vi "Tutorial.vi"() -> ()   [LabVIEW 2016]
panel:
  in  "Set Filter":bool
  out "OptionsFilterFreq2":string[][](array[string])
  out "OptionsFilterFreq1":string[][](array[string])
  in  "Read Filter Options":bool
  in  "3db Frequency #2":u16(ring) items=["100"]
  in  "3dB Frequency #1":u16(ring) items=["10"]
  in  "SampleCount":i64
  out "FilterType":string
  in  "Set Precision":bool
  in  "Precision":i32
  out "Info":string
  out "OptionsArray":string[][](array[string])
  in  "Property":string(combo)
  in  "Options":u16(ring)
  out "VariableInfos":string
  out "SelectedVarID":string
  in  "Write Project To Controller":bool
  in  "Set New Value":bool
  out "ControllerID":string
  in  "ReadOptions":bool
  in  "Network Devices":i32(listbox)=-1
  in  "ScanNetwork":bool
  in  "Variables":i32(listbox)=-1
  in  "ReadVariableIDs":bool
  in  "ReadController":bool
  out "error out":errorcluster
  # "GI.com is used to run a Network-Scan.\nLists all available Gantner-Devices\nin the Network with IP-Address\nand Location."
  # "Upload a device configuration (Q.station) into GI.config for further\nconfiguration. The result (on success) is a valid controller ID (needed \nfor later use)."
  # "Read VariableIDs + Infos from current\nproject in GI.config. IDs are necessary\nfor later use."
  # "Select a Variable to display Infos\nand to do further operations."
  # "This shows a simple example to set 1 variable property directly. \"Precision\" displays the actual setting of the selected variable. Using \"Set Precision\" a new setting can be applied."
  # "Depending on the Type of the selected variable, some more properties can be loaded (also with available options). Here, elements are only visible if an analog input is selected!\n\nUsing this example you can read properties of an analog input (see some examples in the drop-down list), and \"Set\" a new selected value."
  # "Read available options for the selected filter type. Use \"Set Filter\" to apply new settings."
  # "Using \"Write Project\" the current settings are checked for validation and transferred to the controller."
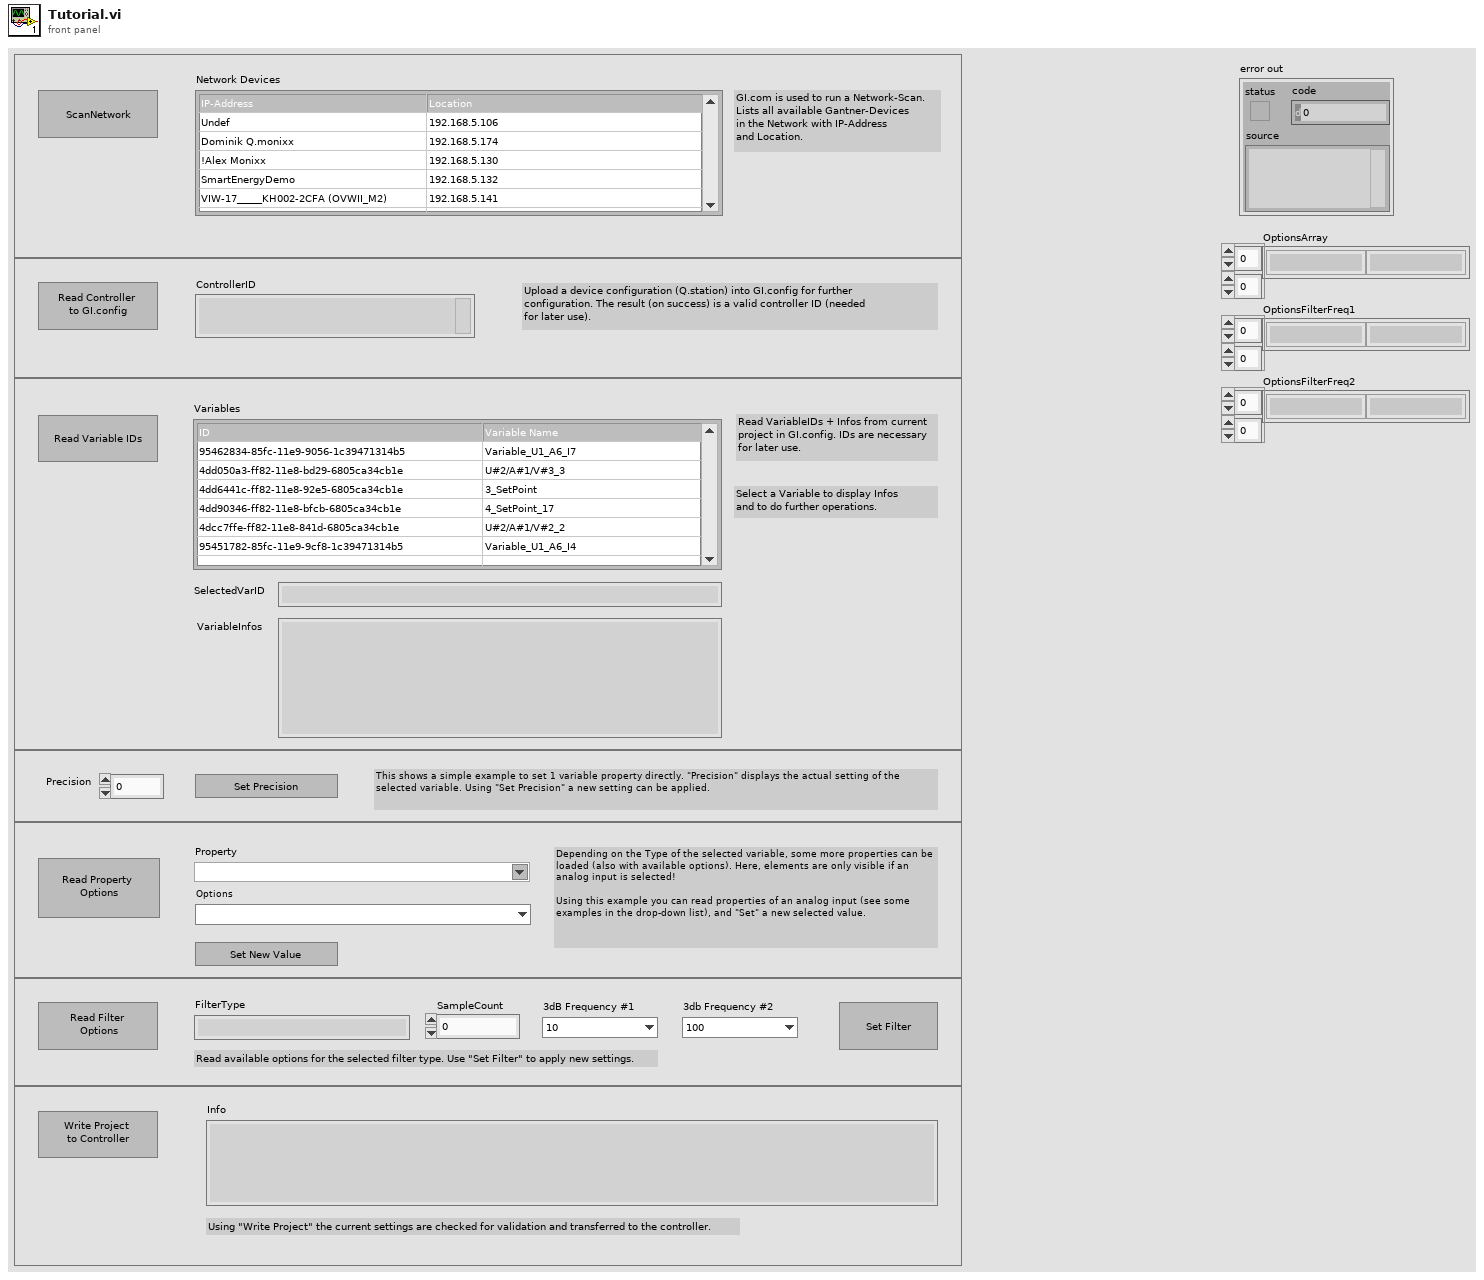
[diagram p1: front panel]
types:
  T1 = enum16{"idle", "idle2", "ScanNetwork", "ReadController", "ReadVarIDs", "ReadOptions", "SetConfig", "WriteToController", "SetPrecision", "ReadFilterOptions", "SetFilter"}
  T2 = enum16{"Bool", "Snippet", "Struct", "Int64", "Int32", "Float", "Double", "String"}
  T3 = typedef "VariableInfo.ctl" = cluster{"Name":string, "ID":string, "Type":string, "DataFormat":string, "DataDirection":string, "OwnerID":string, "AnalogInput Type":string, "Unit":string, "Precision":dbl, "Range":string, "FilterSettings":cluster{"Type":string, "SampleCount":i64, "3dB Frequency #1":string, "3dB Frequency #2":string, "TypeShort":string}}
  T4 = typedef "VariableArray.ctl" = cluster{"Array":T3[]}
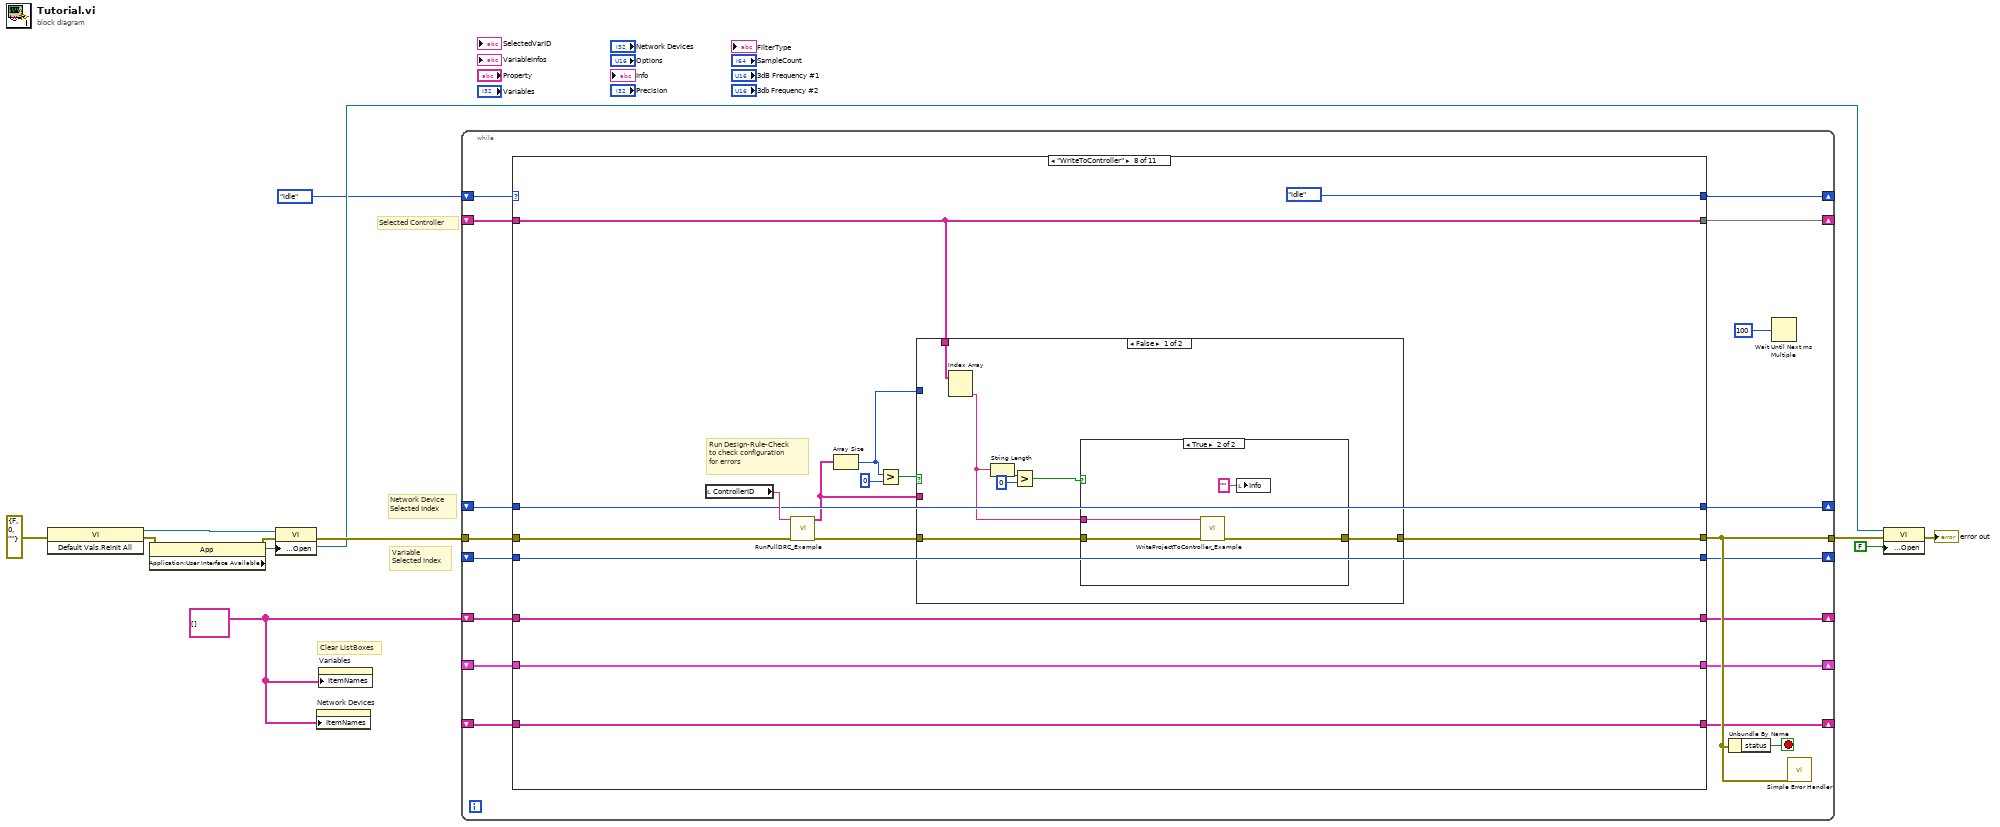
[diagram p0: block diagram]
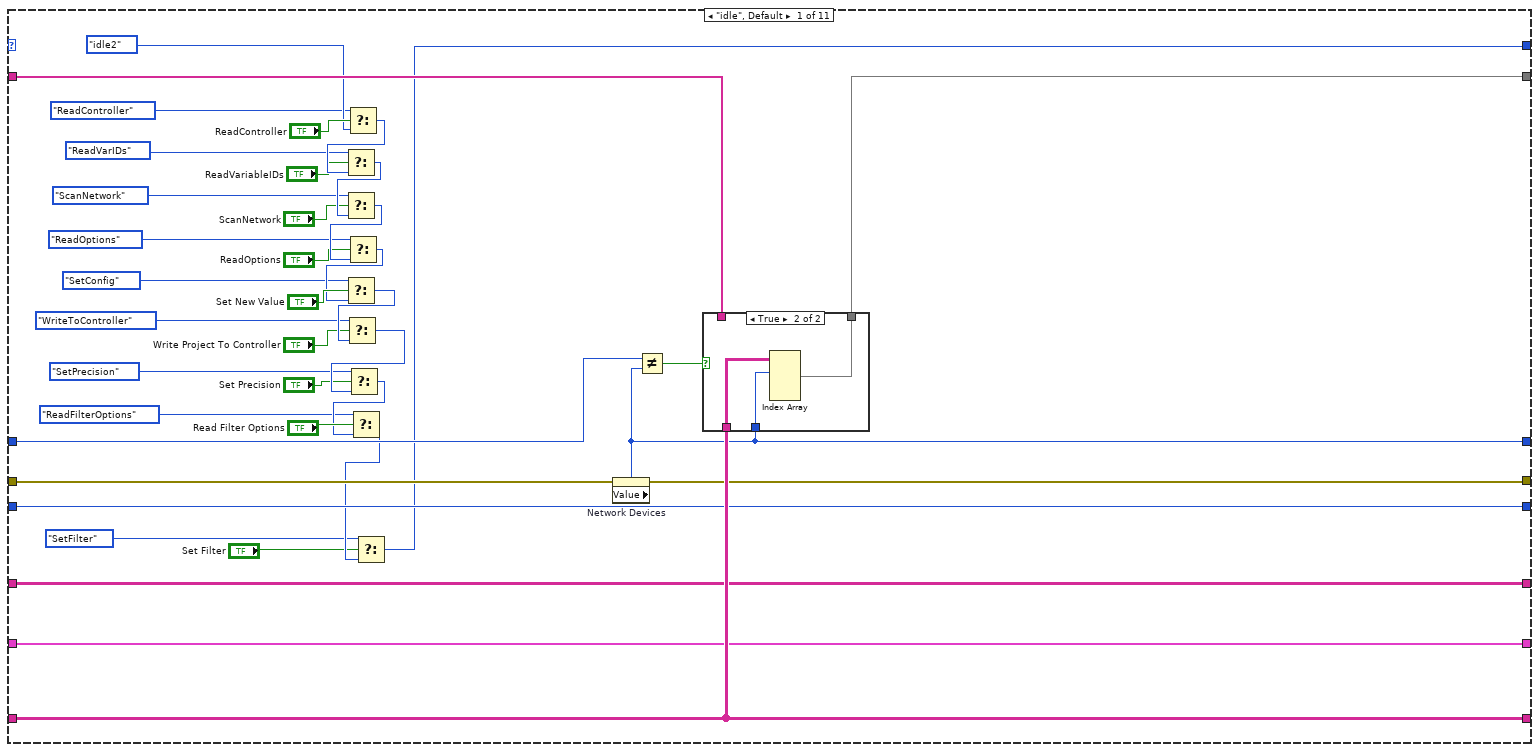
[diagram p2: hidden frame]
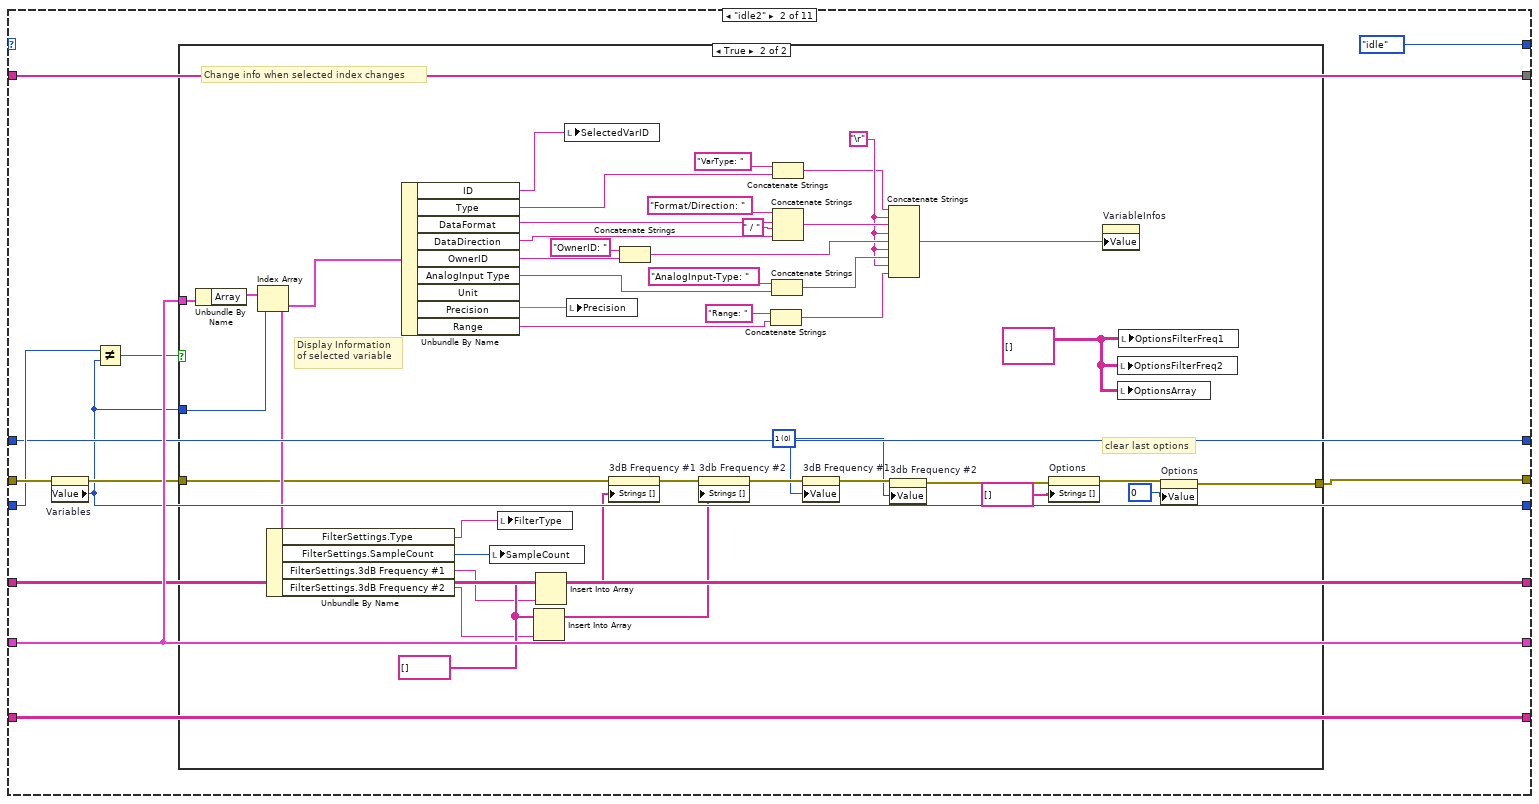
[diagram p4: hidden frame]
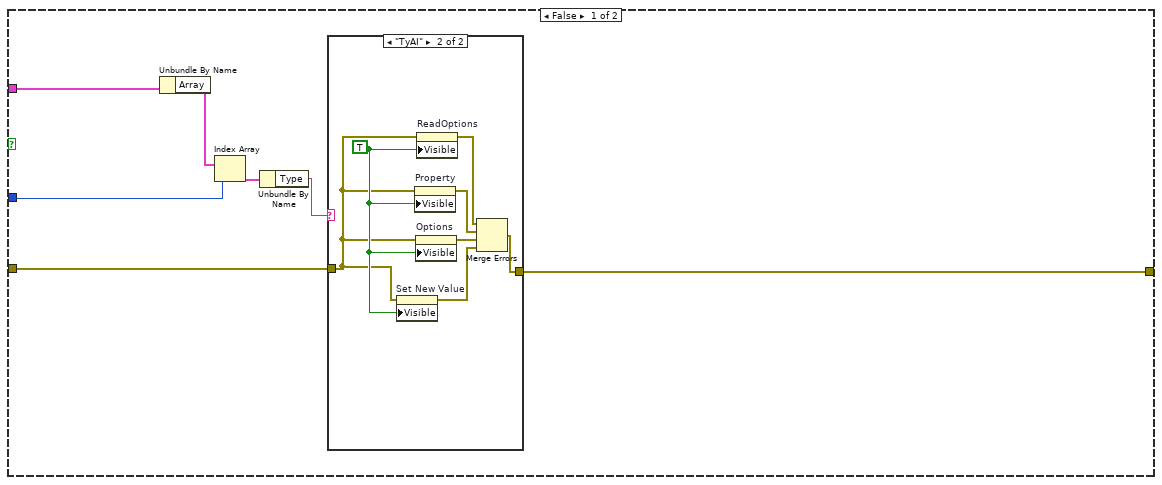
[diagram p5: hidden frame]
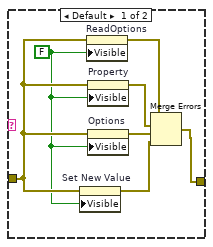
[diagram p6: hidden frame]
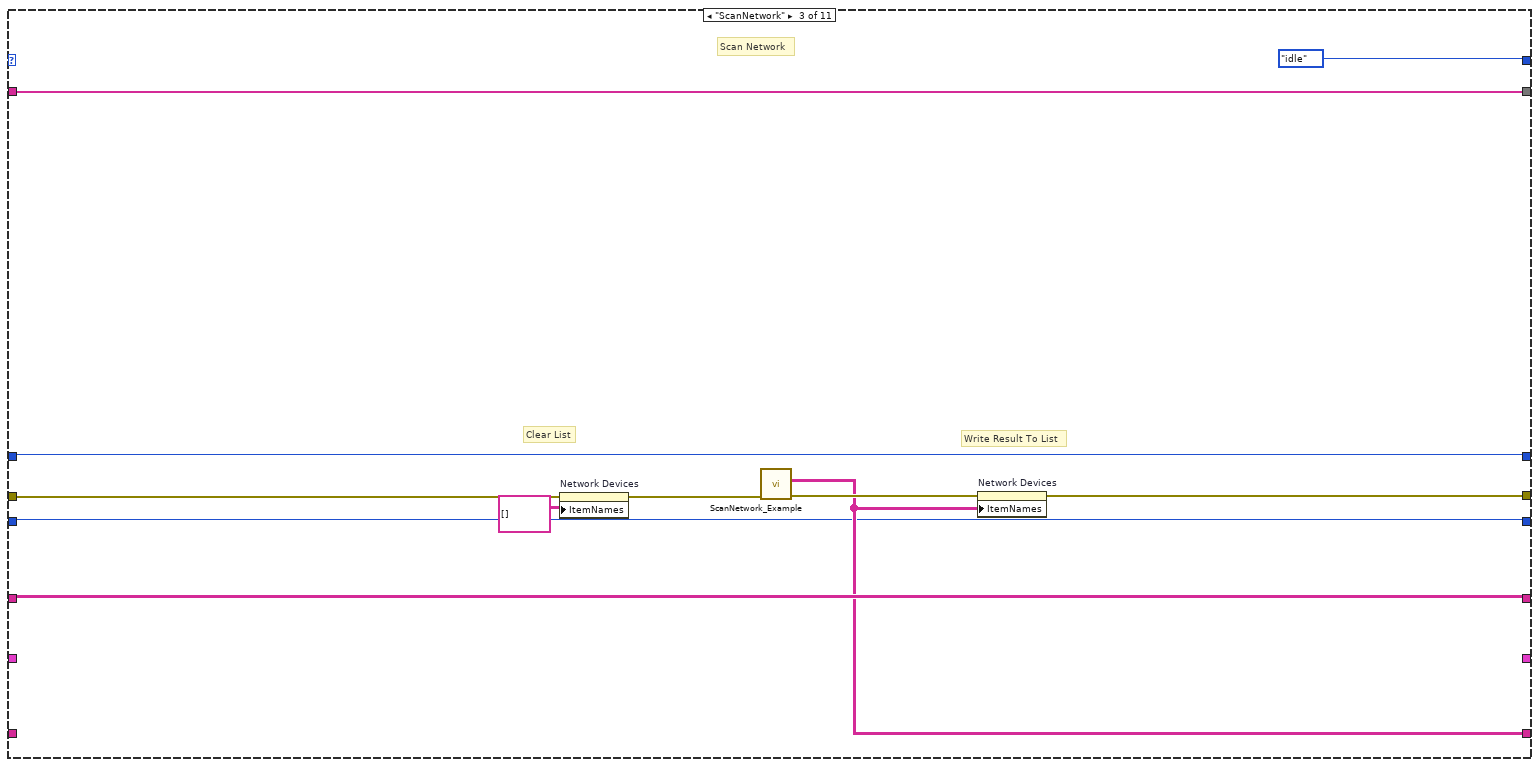
[diagram p7: hidden frame]
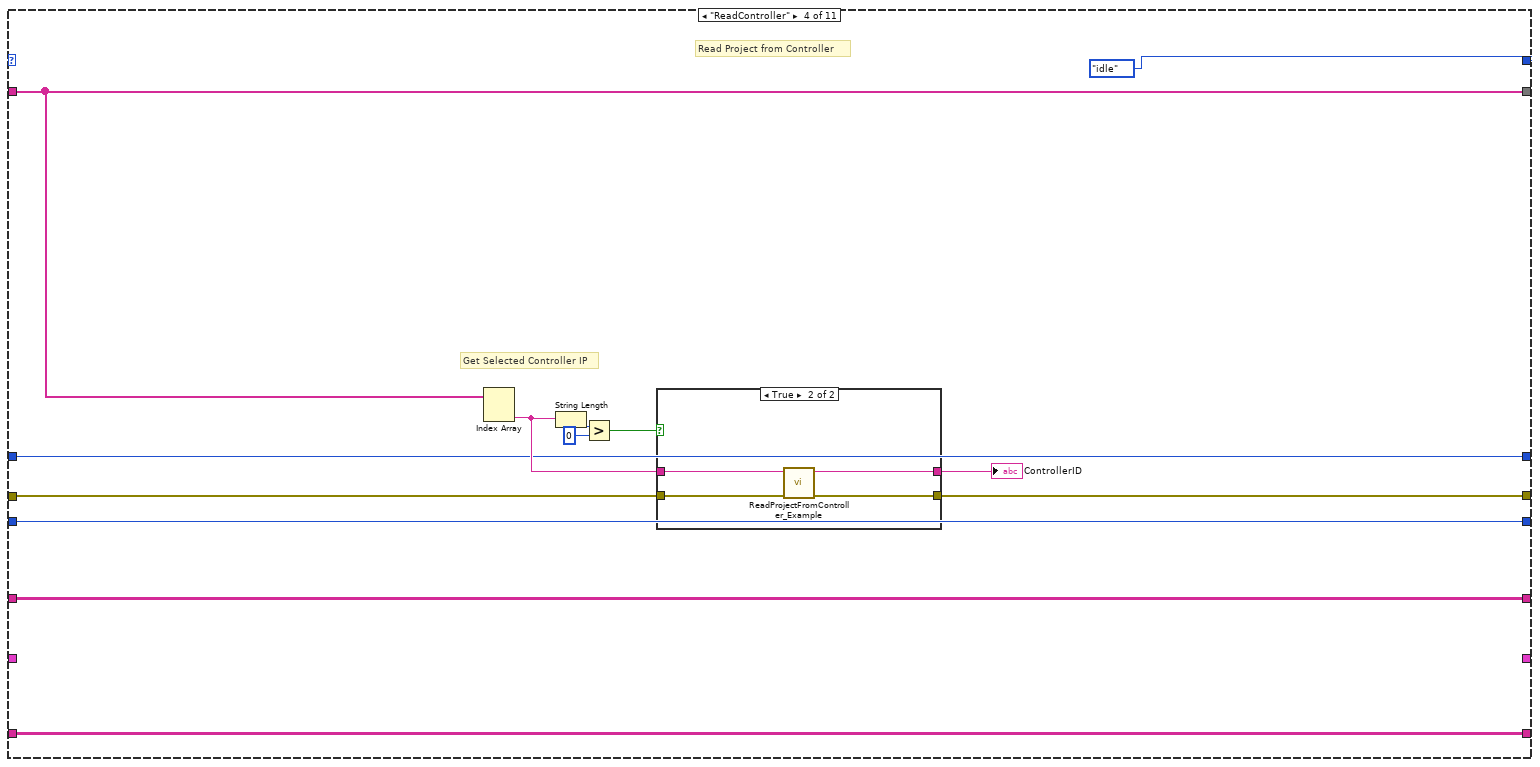
[diagram p8: hidden frame]
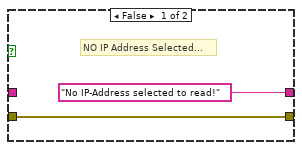
[diagram p9: hidden frame]
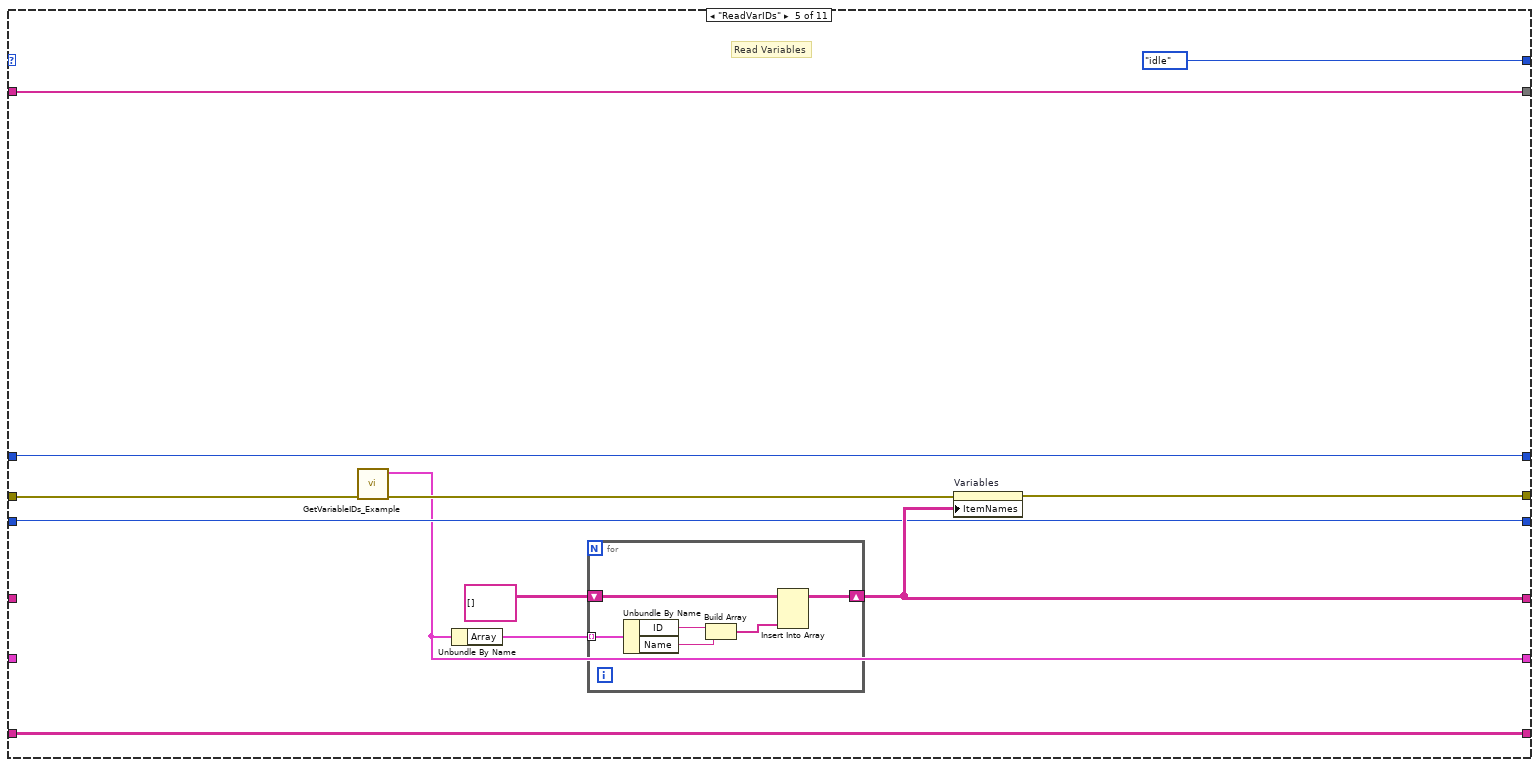
[diagram p10: hidden frame]
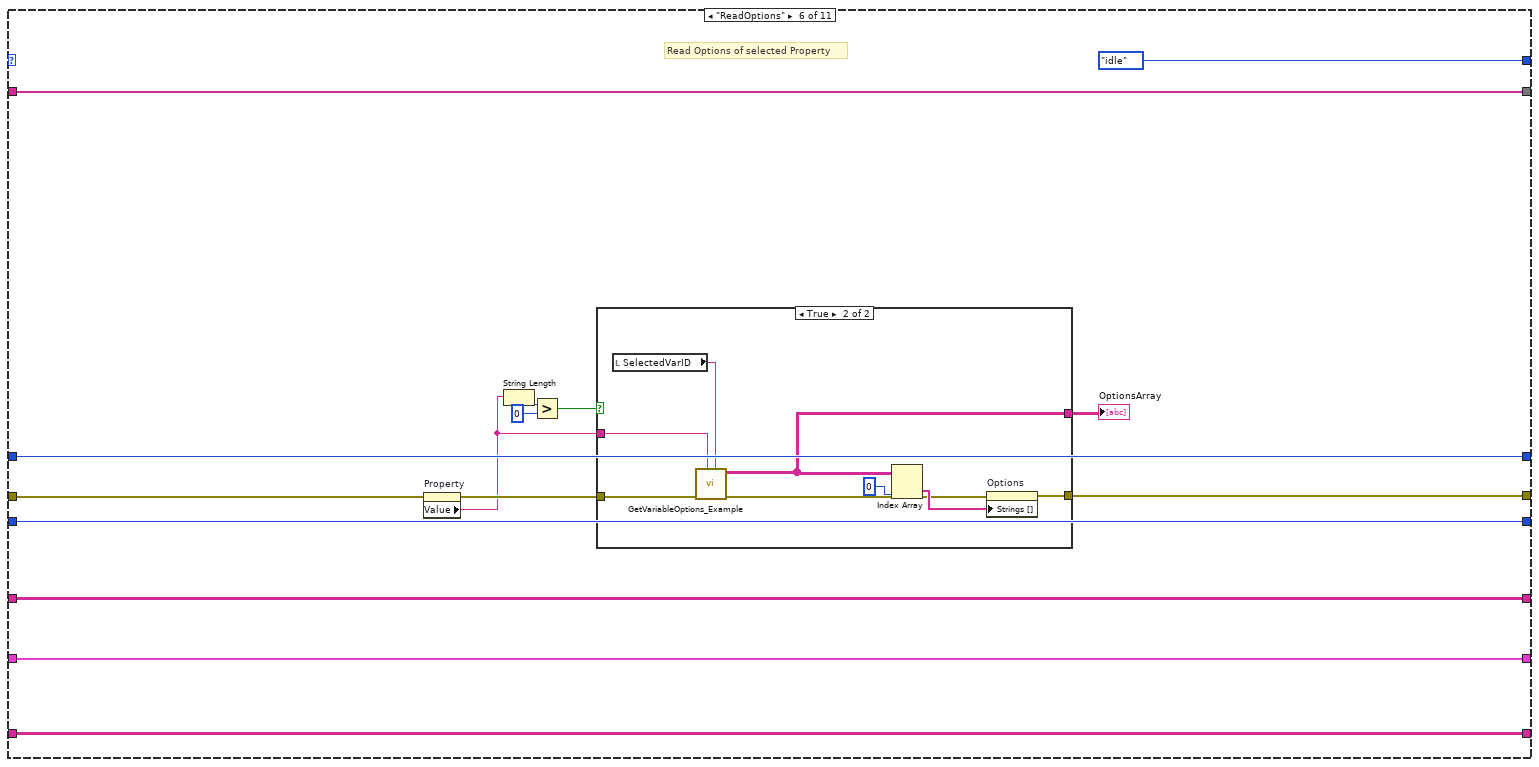
[diagram p11: hidden frame]
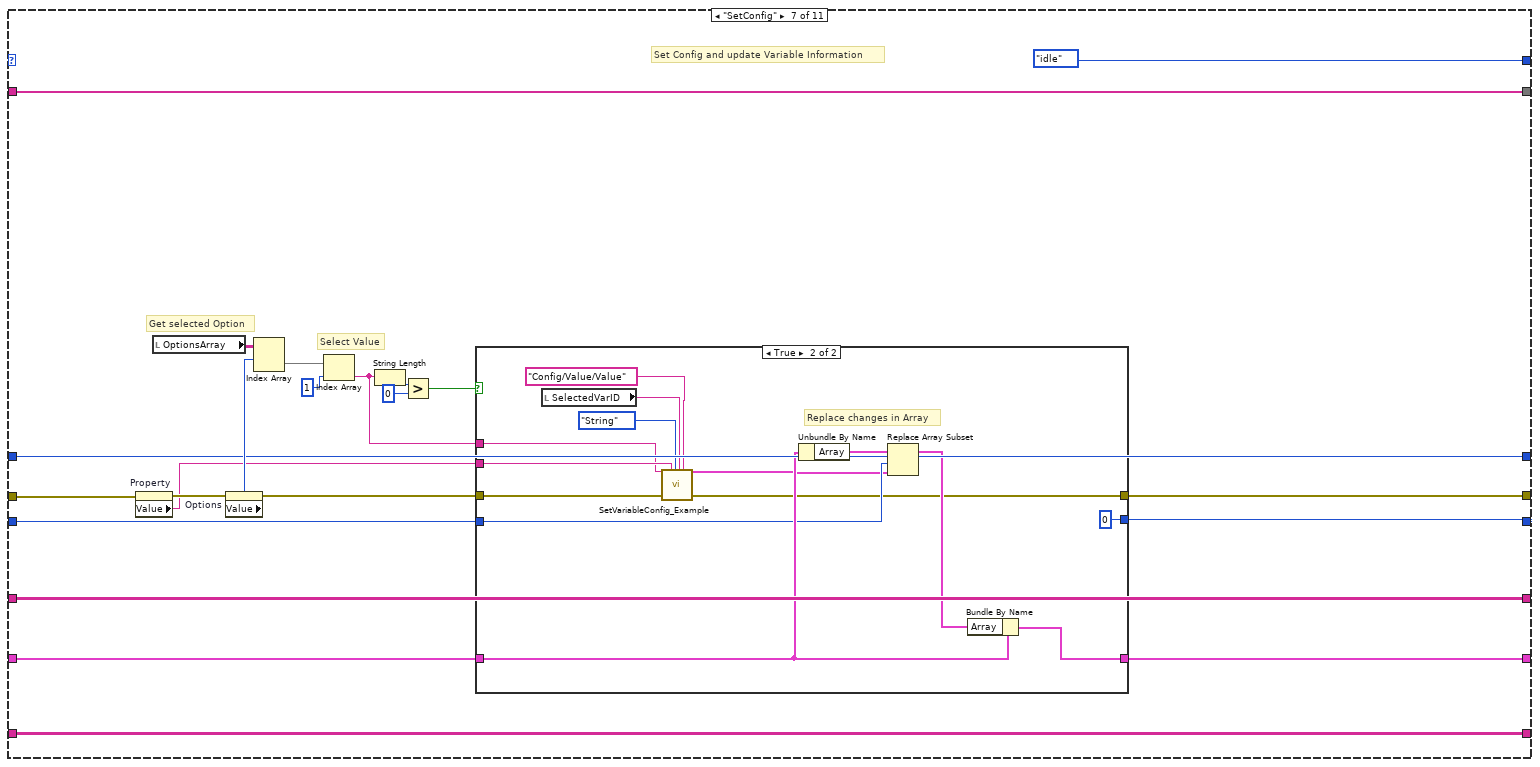
[diagram p13: hidden frame]
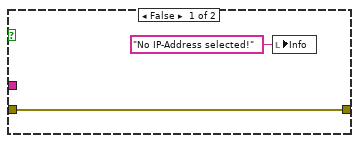
[diagram p15: hidden frame]
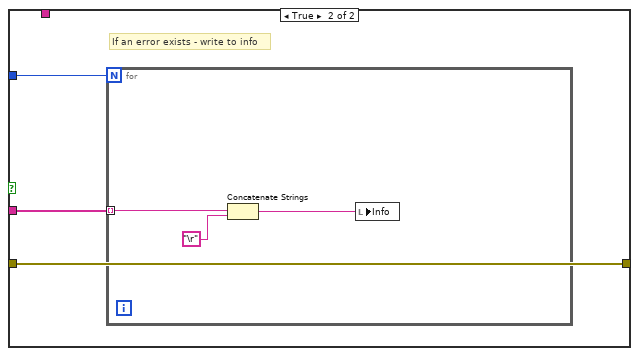
[diagram p16: hidden frame]
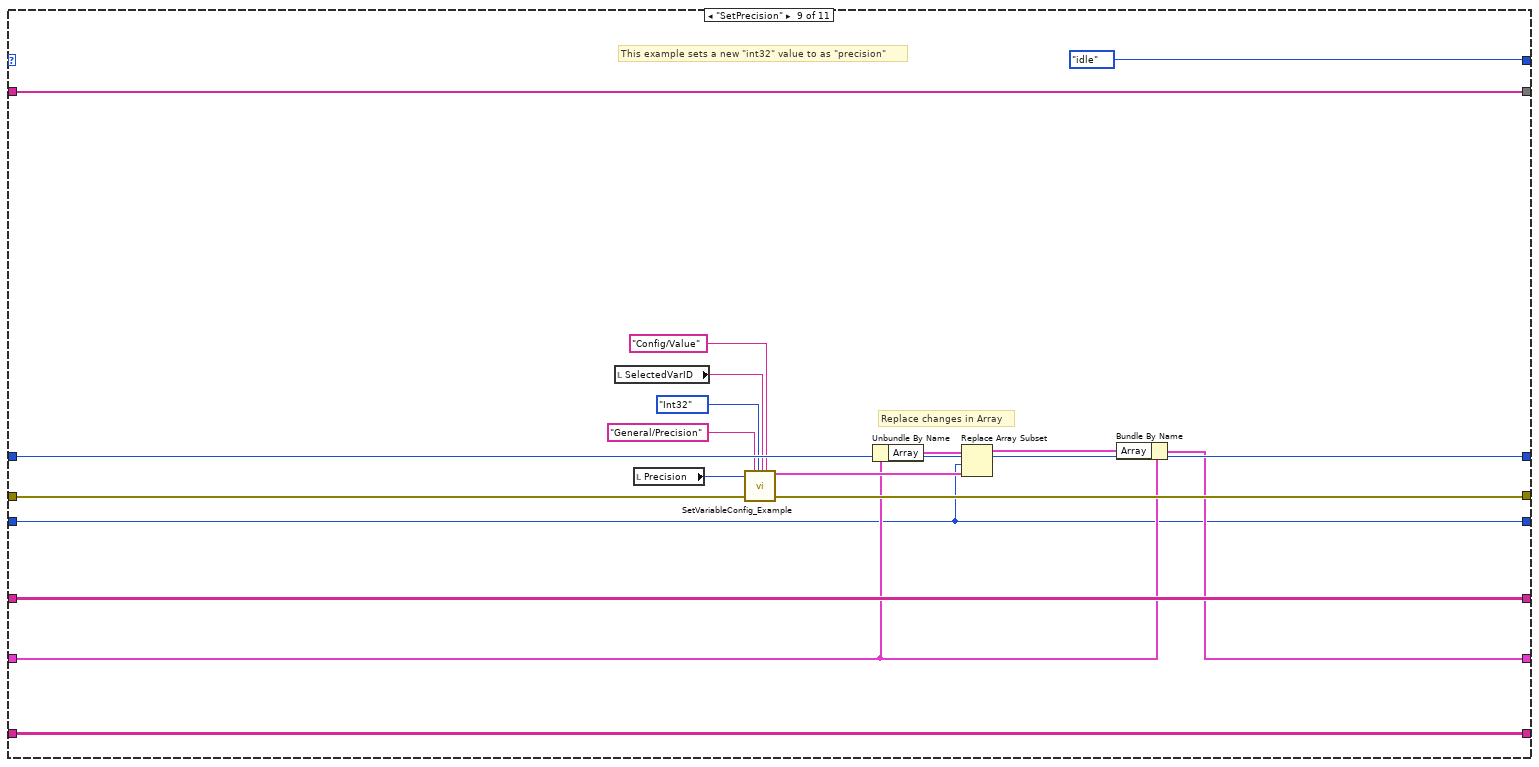
[diagram p17: hidden frame]
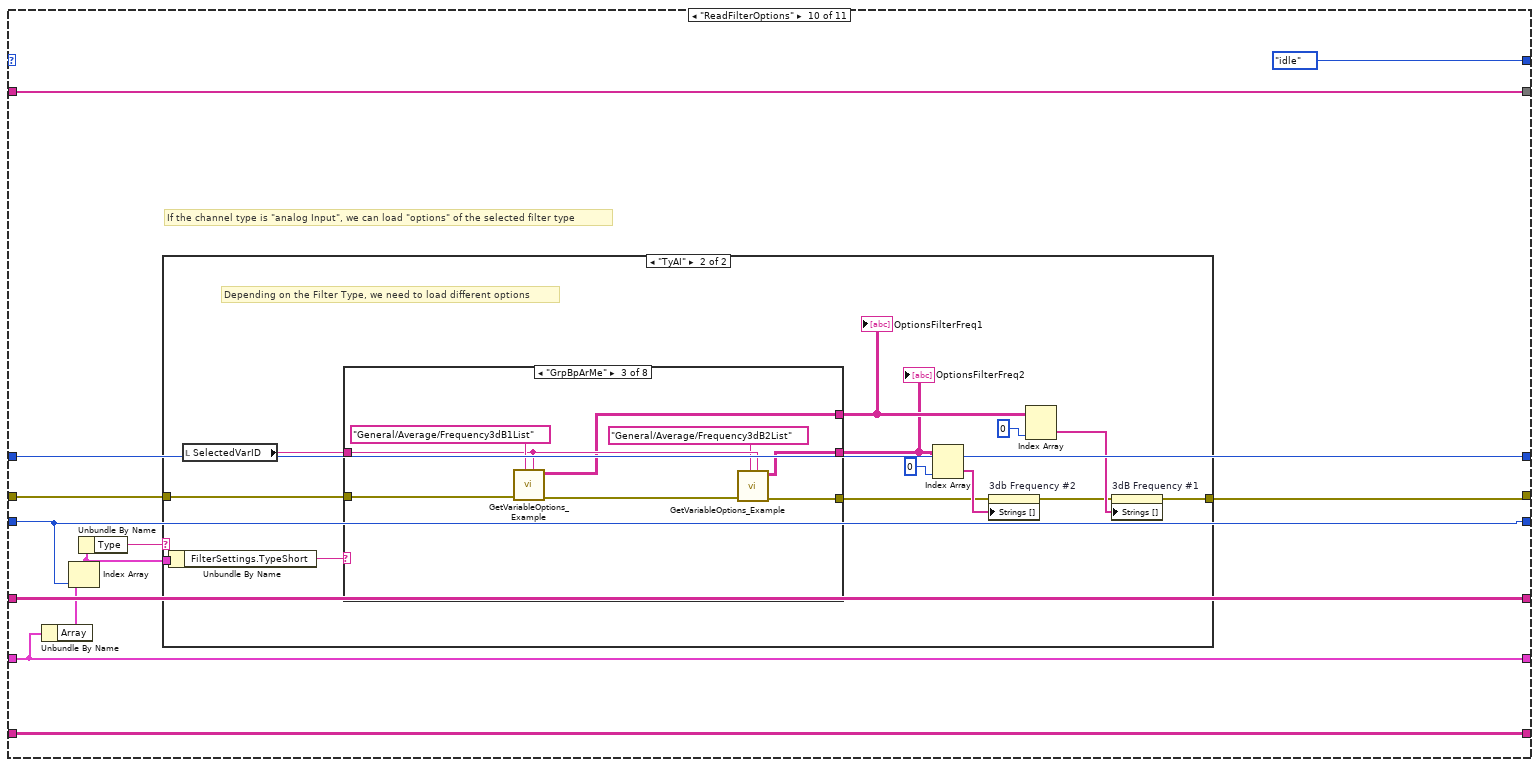
[diagram p18: hidden frame]
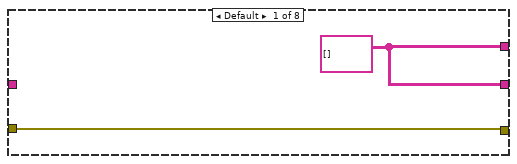
[diagram p20: hidden frame]
diagram:
  w2 = string[][] []
  # "Variable\nSelected Index"
  # "Network Device\nSelected Index"
  # "Selected Controller"
  # "Clear ListBoxes"
  n1 = invoke class="VI" method="Default Vals.Reinit All"(error in=errorcluster {"status"=FALSE, "code"=0, "source"=""} ("Fehler (Eingang, kein Fehler)")) -> (reference out=w12:refnum<vi>, error out=w10:errorcluster)  [unwired: 2 in, 1 out]
  n2 = property class="App"(error in=w10) -> (error out=w9:errorcluster, "Application:User Interface Available"=w11:bool)  [unwired: 1 in, 1 out]
  n3 = property class="VI"(reference=w12, error in=w9, "Front Panel.Open"=w11) -> (reference out=w3:refnum<vi>, error out=w7:errorcluster)
  n4 = property on="Network Devices" class="MCListbox (strict)"("ItemNames"=w2) -> ()  [unwired: 2 in, 2 out]
  n5 = property on="Variables" class="MCListbox (strict)"("ItemNames"=w2) -> ()  [unwired: 2 in, 2 out]
  n6 = while {
    tunnel: w7 -> [w29]
    tunnel: [w28] -> w4
    shift-right: [w14] -> _
    shift-left: T1."idle" -> [w13]
    shift-right: [w26] -> _
    shift-left: w2 -> [w27]
    shift-right: [w24] -> _
    shift-left: _ -> [w25]
    shift-right: [w23] -> _
    shift-left: _ -> [w22]
    shift-right: [w21] -> _
    shift-left: _ -> [w20]
    shift-right: [w19] -> _
    shift-left: _ -> [w18]
    shift-right: [w16] -> _
    shift-left: _ -> [w15]
    stop <- w17 stop-if-true
    n7 = case shown="\"WriteToController\"" w13 {
      tunnel: w29 -> [w64 w85 w156 w173 w190 w207 w237 w275 w308 w315 w389]
      tunnel: [w46 w76 w159 w172 w186 w208 w223 w265 w307 w314 w387] -> w28
      tunnel: w27 -> [w56 w81 w160 w171 _ w212 w242 w273 w310 w323 w394]
      tunnel: [w56 w81 w160 w171 w185 w212 w242 w273 w310 w323 w394] -> w26
      tunnel: w25 -> [w61 w80 _ w170 w191 w211 w243 w272 w309 w324 w395]
      tunnel: [w61 w80 w157 w170 w191 w211 w243 w272 w309 w324 w395] -> w24
      tunnel: [w55 w79 w152 w163 w183 w204 w238 w269 w311 w319 w393] -> w23
      tunnel: w22 -> [w63 w79 w152 w163 w183 w204 w238 w269 w311 w319 w393]
      tunnel: [w60 w78 w151 w162 w181 w203 w239 w264 w312 w318 w392] -> w21
      tunnel: w20 -> [w59 w78 w151 w162 w181 w203 w239 w264 w312 w318 w392]
      tunnel: [w47 w75 w153 w164 w184 w205 w224 w270 w296 w320 0 ("Value")] -> w19
      tunnel: w18 -> [w47 w84 w153 w164 w184 w205 w226 w270 w296 w320 w384]
      tunnel: [w50 w83 _ _ w182 w210 w227 w271 w297 w322 w385] -> w16
      tunnel: w15 -> [w50 w83 _ _ _ w210 w225 w271 w298 w322 w386]
      tunnel: [w33 T1."idle" T1."idle" T1."idle" T1."idle" T1."idle" T1."idle" T1."idle" T1."idle" T1."idle" T1."idle"] -> w14
      frame "idle", Default {
        n8 = Select(t=T1."ReadController", s="ReadController", f=T1."idle2") -> (s? t:f=w68:T1)
        n9 = Select(t=T1."ReadVarIDs", s="ReadVariableIDs", f=w68) -> (s? t:f=w66:T1)
        n10 = Select(t=T1."ScanNetwork", s="ScanNetwork", f=w66) -> (s? t:f=w58:T1)
        n11 = Select(t=T1."ReadOptions", s="ReadOptions", f=w58) -> (s? t:f=w53:T1)
        n12 = Select(t=T1."SetConfig", s="Set New Value", f=w53) -> (s? t:f=w52:T1)
        n13 = Select(t=T1."WriteToController", s="Write Project To Controller", f=w52) -> (s? t:f=w49:T1)
        n14 = Select(t=T1."SetPrecision", s="Set Precision", f=w49) -> (s? t:f=w44:T1)
        n15 = Select(t=T1."ReadFilterOptions", s="Read Filter Options", f=w44) -> (s? t:f=w34:T1)
        n16 = Select(t=T1."SetFilter", s="Set Filter", f=w34) -> (s? t:f=w33:T1)
        n17 = property on="Network Devices" class="MCListbox (strict)"(error in=w64) -> (error out=w46:errorcluster, "Value"=w55:i32)  [unwired: 1 in, 1 out]
        n18 = Not Equal?(x=w63, y=w55) -> (x != y?=w62:bool)
        n19 = case shown="True" w62 {
          tunnel: w55 -> [_ w71]
          tunnel: w61 -> [_ w73]
          tunnel: [w70 w72] -> w60
          tunnel: w59 -> [w70 _]
          frame False {
          }
          frame True {
            n20 = Index Array(array=w73, index (row) #1=w71) -> (element #1=w72:string[])  [unwired: 3 in, 1 out]
          }
        }
      }
      frame "idle2" {
        n21 = property on="Variables" class="MCListbox (strict)"(error in=w85) -> (error out=w77:errorcluster, "Value"=w75:i32)  [unwired: 1 in, 1 out]
        n22 = Not Equal?(x=w84, y=w75) -> (x != y?=w82:bool)
        n23 = case shown="True" w82 {
          tunnel: w75 -> [w90 w149]
          tunnel: w83 -> [w91 w148]
          tunnel: w77 -> [w87 w119]
          tunnel: [w86 w111] -> w76
          frame False {
            n24 = Unbundle By Name(w91) -> ("Array"=w92:T3[])
            n25 = Index Array(array=w92, index=w90) -> (element=w89:T3)
            n26 = Unbundle By Name(w89) -> ("Type"=w88:string)
            n27 = case shown="\"TyAI\"" w88 {
              tunnel: w87 -> [w95 w100]
              tunnel: [w96 w103] -> w86
              frame Default {
                w93 = FALSE ("Visible")
                n28 = property on="Set New Value" class="Bool"(error in=w95, "Visible"=w93) -> (error out=w94:errorcluster)  [unwired: 1 in, 1 out]
                n29 = property on="ReadOptions" class="Bool"(error in=w95, "Visible"=w93) -> (error out=w97:errorcluster)  [unwired: 1 in, 1 out]
                n30 = property on="Property" class="CmbBox"(error in=w95, "Visible"=w93) -> (error out=w98:errorcluster)  [unwired: 1 in, 1 out]
                n31 = property on="Options" class="Ring (strict)"(error in=w95, "Visible"=w93) -> (error out=w99:errorcluster)  [unwired: 1 in, 1 out]
                n32 = Merge Errors(w97, w98, w99, w94) -> (w96:errorcluster)
              }
              frame "TyAI" {
                w102 = TRUE ("Visible")
                n33 = property on="Set New Value" class="Bool"(error in=w100, "Visible"=w102) -> (error out=w101:errorcluster)  [unwired: 1 in, 1 out]
                n34 = property on="Property" class="CmbBox"(error in=w100, "Visible"=w102) -> (error out=w105:errorcluster)  [unwired: 1 in, 1 out]
                n35 = property on="Options" class="Ring (strict)"(error in=w100, "Visible"=w102) -> (error out=w106:errorcluster)  [unwired: 1 in, 1 out]
                n36 = property on="ReadOptions" class="Bool"(error in=w100, "Visible"=w102) -> (error out=w104:errorcluster)  [unwired: 1 in, 1 out]
                n37 = Merge Errors(w104, w105, w106, w101) -> (w103:errorcluster)
              }
            }
          }
          frame True {
            w107 = u16 0 items=["1"] ("3dB Frequency #1")
            w122 = string[] [] ("Strings []")
            w114 = string[][] [] ("Strings []")
            w112 = u16 0 items=[""] ("Options")
            w128 = "\r"
            # "clear last options"
            # "Change info when selected index changes"
            # "Display Information\nof selected variable"
            n38 = Unbundle By Name(w148) -> ("Array"=w147:T3[])
            n39 = Index Array(array=w147, index=w149) -> (element=w143:T3)
            n40 = Unbundle By Name(w143) -> ("FilterSettings.Type"=w124:string, "FilterSettings.SampleCount"=w123:i64, "FilterSettings.3dB Frequency #1"=w121:string, "FilterSettings.3dB Frequency #2"=w120:string)
            n41 = Unbundle By Name(w143) -> ("ID"=w145:string, "Type"=w141:string, "DataFormat"=w139:string, "DataDirection"=w137:string, "OwnerID"=w135:string, "AnalogInput Type"=w131:string, "Precision"=w144:dbl, "Range"=w126:string)  [unwired: 1 out]
            n42 = local write "SampleCount"(w123) -> ()
            n43 = local write "FilterType"(w124) -> ()
            n44 = Insert Into Array(array=w122, new element=w120) -> (w116:string[])  [unwired: 1 in]
            n45 = Insert Into Array(array=w122, new element=w121) -> (w117:string[])  [unwired: 1 in]
            n46 = local write "SelectedVarID"(w145) -> ()
            n47 = local write "Precision"(w144) -> ()
            n48 = property on="3dB Frequency #1" class="Ring (strict)"(error in=w119, "Strings []"=w117) -> (error out=w118:errorcluster)  [unwired: 1 in, 1 out]
            n49 = Concatenate Strings("OwnerID: " ("string"), w135) -> (w133:string)
            n50 = property on="3db Frequency #2" class="Ring (strict)"(error in=w118, "Strings []"=w116) -> (error out=w110:errorcluster)  [unwired: 1 in, 1 out]
            n51 = Concatenate Strings("Range: " ("string"), w126) -> (w125:string)
            n52 = Concatenate Strings("AnalogInput-Type: " ("string"), w131) -> (w130:string)
            n53 = Concatenate Strings("VarType: " ("string"), w141) -> (w115:string)
            n54 = Concatenate Strings("Format/Direction: " ("string"), w139, " / " ("string"), w137) -> (w134:string)
            n55 = property on="3dB Frequency #1" class="Ring (strict)"(error in=w110, "Value"=w107) -> (error out=w109:errorcluster)  [unwired: 1 in, 1 out]
            n56 = Concatenate Strings(w115, w128, w134, w128, w133, w128, w130, w128, w125) -> (w129:string)
            n57 = property on="3db Frequency #2" class="Ring (strict)"(error in=w109, "Value"=w107) -> (error out=w108:errorcluster)  [unwired: 1 in, 1 out]
            n58 = property on="Options" class="Ring (strict)"(error in=w108, "Strings []"=string[] []) -> (error out=w146:errorcluster)  [unwired: 1 in, 1 out]
            n59 = property on="VariableInfos" class="Str"("Value"=w129) -> ()  [unwired: 2 in, 2 out]
            n60 = local write "OptionsFilterFreq2"(w114) -> ()
            n61 = local write "OptionsArray"(w114) -> ()
            n62 = local write "OptionsFilterFreq1"(w114) -> ()
            n63 = property on="Options" class="Ring (strict)"(error in=w146, "Value"=w112) -> (error out=w111:errorcluster)  [unwired: 1 in, 1 out]
          }
        }
      }
      frame "ScanNetwork" {
        # "Write Result To List"
        # "Clear List"
        # "Scan Network"
        n64 = property on="Network Devices" class="MCListbox (strict)"(error in=w156, "ItemNames"=string[][] [] ("Item Names")) -> (error out=w155:errorcluster)  [unwired: 1 in, 1 out]
        n65 = call "ScanNetwork_Example.vi"("Fehler (Eingang, kein Fehler)"=w155) -> ("Fehler (Ausgang)"=w158:errorcluster, "NetworkDevices Array"=w157:string[][])  [unwired: 9 in]
        n66 = property on="Network Devices" class="MCListbox (strict)"(error in=w158, "ItemNames"=w157) -> (error out=w159:errorcluster)  [unwired: 1 in, 1 out]
      }
      frame "ReadController" {
        # "Get Selected Controller IP"
        # "Read Project from Controller"
        n67 = Index Array(array=w162) -> (element #2=w165:string)  [unwired: 2 in, 1 out]
        n68 = String Length(string=w165) -> (length=w169:i32)
        n69 = Greater?(x=w169, y=0) -> (0:w167:bool)
        n70 = case shown="True" w167 {
          tunnel: w173 -> [w175 w179]
          tunnel: [w175 w178] -> w172
          tunnel: w165 -> [_ w177]
          tunnel: ["No IP-Address selected to read!" ("standard output") w176] -> w166
          frame False {
            # "NO IP Address Selected..."
          }
          frame True {
            n71 = call "ReadProjectFromController_Example.vi"("Fehler (Eingang, kein Fehler)"=w179, "ControllerIP"=w177) -> ("Fehler (Ausgang)"=w178:errorcluster, "ControllerID"=w176:string)  [unwired: 8 in]
          }
        }
        "ControllerID" <- w166
      }
      frame "ReadVarIDs" {
        # "Read Variables"
        n72 = call "GetVariableIDs_Example.vi"("Fehler (Eingang, kein Fehler)"=w190) -> ("Fehler (Ausgang)"=w189:errorcluster, "VariableArray out"=w182:T4)  [unwired: 9 in]
        n73 = Unbundle By Name(w182) -> ("Array"=w188:T3[])
        n74 = for {
          tunnel: w188 -> [w197] mode=indexing
          shift-right: [w195] -> w185
          shift-left: string[][] [] ("Item Names") -> [w196]
          n75 = Unbundle By Name(w197) -> ("ID"=w194:string, "Name"=w193:string)
          n76 = Build Array(w194, w193) -> (w192:string[])
          n77 = Insert Into Array(array=w196, new element=w192) -> (w195:string[][])  [unwired: 2 in]
        }
        n78 = property on="Variables" class="MCListbox (strict)"(error in=w189, "ItemNames"=w185) -> (error out=w186:errorcluster)  [unwired: 1 in, 1 out]
      }
      frame "ReadOptions" {
        # "Read Options of selected Property"
        n79 = property on="Property" class="CmbBox"(error in=w207) -> (error out=w206:errorcluster, "Value"=w199:string)  [unwired: 1 in, 1 out]
        n80 = String Length(string=w199) -> (length=w202:i32)
        n81 = Greater?(x=w202, y=0) -> (0:w200:bool)
        n82 = case shown="True" w200 {
          tunnel: [_ w221] -> w209
          tunnel: [w213 w217] -> w208
          tunnel: w206 -> [w213 w216]
          tunnel: w199 -> [_ w215]
          frame False {
          }
          frame True {
            n83 = local read "SelectedVarID"() -> (w214:string)
            n84 = call "GetVariableOptions_Example.vi"("VariableID"=w214, "PropertyName"=w215, "Fehler (Eingang, kein Fehler)"=w216) -> ("Fehler (Ausgang)"=w218:errorcluster, "Options"=w221:string[][])  [unwired: 7 in]
            n85 = Index Array(array=w221, index (col)=0 ("disabled index (col)")) -> (element=w219:string[])  [unwired: 1 in]
            n86 = property on="Options" class="Ring (strict)"(error in=w218, "Strings []"=w219) -> (error out=w217:errorcluster)  [unwired: 1 in, 1 out]
          }
        }
        "OptionsArray" <- w209
      }
      frame "SetConfig" {
        # "Set Config and update Variable Information"
        # "Select Value"
        # "Get selected Option"
        n87 = property on="Property" class="CmbBox"(error in=w237) -> (error out=w236:errorcluster, "Value"=w228:string)  [unwired: 1 in, 1 out]
        n88 = local read "OptionsArray"() -> (w241:string[][])
        n89 = property on="Options" class="Ring (strict)"(error in=w236) -> (error out=w230:errorcluster, "Value"=w240:u16)  [unwired: 1 in, 1 out]
        n90 = Index Array(array=w241, index (row)=w240) -> (element=w233:string[])  [unwired: 1 in]
        n91 = Index Array(array=w233, index=1) -> (element=w229:string)
        n92 = String Length(string=w229) -> (length=w235:i32)
        n93 = Greater?(x=w235, y=0) -> (0:w232:bool)
        n94 = case shown="True" w232 {
          tunnel: w230 -> [w246 w253]
          tunnel: [w246 w254] -> w223
          tunnel: w229 -> [_ w250]
          tunnel: w228 -> [_ w252]
          tunnel: [w244 w258] -> w227
          tunnel: w226 -> [w245 w256]
          tunnel: w225 -> [w244 w257]
          tunnel: [w245 0 ("Value")] -> w224
          frame False {
          }
          frame True {
            # "Replace changes in Array"
            n95 = local read "SelectedVarID"() -> (w251:string)
            n96 = call "SetVariableConfig_Example.vi"("StringValue or Snippet 2"=w250, "Fehler (Eingang, kein Fehler)"=w253, "PropertyName"=w252, "DataType"=T2."String", "VariableID"=w251, "ConfigMemberName"="Config/Value/Value" ("MemberName")) -> ("VariableInfo out"=w255:T3, "Fehler (Ausgang)"=w254:errorcluster)  [unwired: 20 in]
            n97 = Unbundle By Name(w257) -> ("Array"=w260:T3[])
            n98 = Replace Array Subset(array=w260, new element=w255, index=w256) -> (w259:T3[])
            n99 = Bundle By Name(cluster=w257, "Array"=w259) -> (w258:T4)
          }
        }
      }
      frame "WriteToController" {
        # "Run Design-Rule-Check\nto check configuration\nfor errors"
        n100 = local read "ControllerID"() -> (w274:string)
        n101 = call "RunFullDRC_Example.vi"("Fehler (Eingang, kein Fehler)"=w275, "ControllerID"=w274) -> ("Fehler (Ausgang)"=w266:errorcluster, "Results"=w262:string[])  [unwired: 8 in]
        n102 = Array Size(array=w262) -> (size(s)=w263:i32)
        n103 = Greater?(x=w263, y=0) -> (0:w267:bool)
        n104 = case shown="False" w267 {
          tunnel: w266 -> [w282 w291]
          tunnel: [w281 w291] -> w265
          tunnel: w264 -> [w280 _]
          tunnel: w263 -> [_ w290]
          tunnel: w262 -> [_ w289]
          frame False {
            n105 = Index Array(array=w280) -> (element #2=w276:string)  [unwired: 2 in, 1 out]
            n106 = String Length(string=w276) -> (length=w279:i32)
            n107 = Greater?(x=w279, y=0) -> (0:w277:bool)
            n108 = case shown="True" w277 {
              tunnel: w282 -> [w284 w288]
              tunnel: [w284 w287] -> w281
              tunnel: w276 -> [_ w286]
              frame False {
                n109 = local write "Info"("No IP-Address selected!" ("Info")) -> ()
              }
              frame True {
                n110 = call "WriteProjectToController_Example.vi"("Fehler (Eingang, kein Fehler)"=w288, "Controller IP"=w286) -> ("Fehler (Ausgang)"=w287:errorcluster)  [unwired: 9 in]
                n111 = local write "Info"("" ("Info")) -> ()
              }
            }
          }
          frame True {
            # "If an error exists - write to info"
            n112 = for {
              N: w290 -> [_]
              tunnel: w289 -> [w294] mode=indexing
              n113 = Concatenate Strings(w294, "\r") -> (w292:string)
              n114 = local write "Info"(w292) -> ()
            }
          }
        }
      }
      frame "SetPrecision" {
        # "This example sets a new \"int32\" value to as \"precision\""
        # "Replace changes in Array"
        n115 = local read "SelectedVarID"() -> (w306:string)
        n116 = local read "Precision"() -> (w304:i32)
        n117 = call "SetVariableConfig_Example.vi"("Int32Value or struct"=w304, "Fehler (Eingang, kein Fehler)"=w308, "PropertyName"="General/Precision", "DataType"=T2."Int32", "VariableID"=w306, "ConfigMemberName"="Config/Value" ("MemberName")) -> ("VariableInfo out"=w300:T3, "Fehler (Ausgang)"=w307:errorcluster)  [unwired: 20 in]
        n118 = Unbundle By Name(w298) -> ("Array"=w301:T3[])
        n119 = Replace Array Subset(array=w301, new element=w300, index=w296) -> (w299:T3[])
        n120 = Bundle By Name(cluster=w298, "Array"=w299) -> (w297:T4)
      }
      frame "ReadFilterOptions" {
        # "If the channel type is \"analog Input\", we can load \"options\" of the selected filter type"
        n121 = Unbundle By Name(w322) -> ("Array"=w321:T3[])
        n122 = Index Array(array=w321, index=w320) -> (element=w316:T3)
        n123 = Unbundle By Name(w316) -> ("Type"=w317:string)
        n124 = case shown="\"TyAI\"" w317 {
          tunnel: w316 -> [_ w337]
          tunnel: w315 -> [w325 w335]
          tunnel: [w325 w326] -> w314
          frame Default {
          }
          frame "TyAI" {
            # "Depending on the Filter Type, we need to load different options"
            n125 = Unbundle By Name(w337) -> ("FilterSettings.TypeShort"=w336:string)
            n126 = local read "SelectedVarID"() -> (w338:string)
            n127 = case shown="\"GrpBpArMe\"" w336 {
              tunnel: w338 -> [_ _ w346 w355 w360 w365 w371 w375]
              tunnel: w335 -> [w340 w342 w350 w354 w362 w367 w373 w380]
              tunnel: [w340 w342 w347 w353 w359 w366 w372 w378] -> w328
              tunnel: [w339 w341 w344 string[][] [] ("Options") string[][] [] ("Options") string[][] [] ("Options") string[][] [] ("Options") w377] -> w331
              tunnel: [w339 w341 w343 w352 w358 w363 w370 w376] -> w332
              frame Default {
                w339 = string[][] [] ("Options")
              }
              frame "GrpNo" {
                w341 = string[][] [] ("Options")
              }
              frame "GrpBpArMe" {
                n128 = call "GetVariableOptions_Example.vi"("VariableID"=w346, "PropertyName"="General/Average/Frequency3dB1List", "Fehler (Eingang, kein Fehler)"=w350) -> ("Fehler (Ausgang)"=w348:errorcluster, "Options"=w343:string[][])  [unwired: 7 in]
                n129 = call "GetVariableOptions_Example.vi"("VariableID"=w346, "PropertyName"="General/Average/Frequency3dB2List", "Fehler (Eingang, kein Fehler)"=w348) -> ("Fehler (Ausgang)"=w347:errorcluster, "Options"=w344:string[][])  [unwired: 7 in]
              }
              frame "GrpHp" {
                n130 = call "GetVariableOptions_Example.vi"("VariableID"=w355, "PropertyName"="General/Average/Frequency3dB1List", "Fehler (Eingang, kein Fehler)"=w354) -> ("Fehler (Ausgang)"=w353:errorcluster, "Options"=w352:string[][])  [unwired: 7 in]
              }
              frame "GrpHpArMe" {
                n131 = call "GetVariableOptions_Example.vi"("VariableID"=w360, "PropertyName"="General/Average/Frequency3dB1List", "Fehler (Eingang, kein Fehler)"=w362) -> ("Fehler (Ausgang)"=w359:errorcluster, "Options"=w358:string[][])  [unwired: 7 in]
              }
              frame "GrpLp" {
                n132 = call "GetVariableOptions_Example.vi"("VariableID"=w365, "PropertyName"="General/Average/Frequency3dB1List", "Fehler (Eingang, kein Fehler)"=w367) -> ("Fehler (Ausgang)"=w366:errorcluster, "Options"=w363:string[][])  [unwired: 7 in]
              }
              frame "GrpLpArMe" {
                n133 = call "GetVariableOptions_Example.vi"("VariableID"=w371, "PropertyName"="General/Average/Frequency3dB1List", "Fehler (Eingang, kein Fehler)"=w373) -> ("Fehler (Ausgang)"=w372:errorcluster, "Options"=w370:string[][])  [unwired: 7 in]
              }
              frame "GrpBp" {
                n134 = call "GetVariableOptions_Example.vi"("VariableID"=w375, "PropertyName"="General/Average/Frequency3dB1List", "Fehler (Eingang, kein Fehler)"=w380) -> ("Fehler (Ausgang)"=w379:errorcluster, "Options"=w376:string[][])  [unwired: 7 in]
                n135 = call "GetVariableOptions_Example.vi"("VariableID"=w375, "PropertyName"="General/Average/Frequency3dB2List", "Fehler (Eingang, kein Fehler)"=w379) -> ("Fehler (Ausgang)"=w378:errorcluster, "Options"=w377:string[][])  [unwired: 7 in]
              }
            }
            "OptionsFilterFreq1" <- w332
            "OptionsFilterFreq2" <- w331
            n136 = Index Array(array=w331, index (col)=0 ("disabled index (col)")) -> (element=w330:string[])  [unwired: 1 in]
            n137 = property on="3db Frequency #2" class="Ring (strict)"(error in=w328, "Strings []"=w330) -> (error out=w327:errorcluster)  [unwired: 1 in, 1 out]
            n138 = Index Array(array=w332, index (col)=0 ("disabled index (col)")) -> (element=w329:string[])  [unwired: 1 in]
            n139 = property on="3dB Frequency #1" class="Ring (strict)"(error in=w327, "Strings []"=w329) -> (error out=w326:errorcluster)  [unwired: 1 in, 1 out]
          }
        }
      }
      frame "SetFilter" {
        # "Filter Settings are only available for Variables of Type \"Analog Input\""
        n140 = Unbundle By Name(w386) -> ("Array"=w396:T3[])
        n141 = Index Array(array=w396, index=w384) -> (element=w388:T3)
        n142 = Unbundle By Name(w388) -> ("Type"=w390:string)
        n143 = case shown="\"TyAI\"" w390 {
          tunnel: w388 -> [_ w421]
          tunnel: w389 -> [w398 w418]
          tunnel: [w398 w405] -> w387
          tunnel: w386 -> [w397 w399]
          tunnel: [w397 w401] -> w385
          tunnel: w384 -> [_ w400]
          frame Default {
          }
          frame "TyAI" {
            # "replace information in array"
            # "Get selected option"
            # "Select Value"
            # "Depending on the Filter Type, we need to set different options"
            n144 = local read "OptionsFilterFreq1"() -> (w413:string[][])
            n145 = property on="3dB Frequency #1" class="Ring (strict)"(error in=w418) -> (error out=w417:errorcluster, "Value"=w412:u16)  [unwired: 1 in, 1 out]
            n146 = Index Array(array=w413, index (row)=w412) -> (element=w415:string[])  [unwired: 1 in]
            n147 = Index Array(array=w415, index=1) -> (element=w411:string)
            n148 = local read "OptionsFilterFreq2"() -> (w409:string[][])
            n149 = property on="3db Frequency #2" class="Ring (strict)"(error in=w417) -> (error out=w416:errorcluster, "Value"=w410:u16)  [unwired: 1 in, 1 out]
            n150 = Unbundle By Name(w421) -> ("FilterSettings.TypeShort"=w420:string)
            n151 = Index Array(array=w409, index (row)=w410) -> (element=w407:string[])  [unwired: 1 in]
            n152 = local read "SelectedVarID"() -> (w419:string)
            n153 = Index Array(array=w407, index=1) -> (element=w406:string)
            n154 = case shown="\"GrpBpArMe\"" w420 {
              tunnel: w419 -> [_ _ w436 w469 w493 w521 w544 w577]
              tunnel: w416 -> [w426 w431 w437 w471 w494 w522 w545 w578]
              tunnel: [w426 w431 w433 w470 w492 w520 w543 w576] -> w405
              tunnel: w411 -> [_ _ w434 w466 w489 w516 w540 w568]
              tunnel: w406 -> [_ _ w435 _ _ _ _ w567]
              tunnel: [w422 w427 w432 w464 w487 w515 w538 w566] -> w403
              tunnel: w400 -> [w423 w428 _ w463 w485 w513 w536 w564]
              tunnel: w399 -> [w424 w429 _ w462 w486 w514 w537 w565]
              frame Default {
                # "wirte old value"
                n155 = Unbundle By Name(w424) -> ("Array"=w425:T3[])
                n156 = Index Array(array=w425, index=w423) -> (element=w422:T3)
              }
              frame "GrpNo" {
                # "No Filter"
                # "wirte old value"
                n157 = Unbundle By Name(w429) -> ("Array"=w430:T3[])
                n158 = Index Array(array=w430, index=w428) -> (element=w427:T3)
              }
              frame "GrpBpArMe" {
                # "Bandpass and Arithmetic mean"
                # "Check if string is not empty"
                n159 = String Length(string=w434) -> (length=w444:i32)
                n160 = String Length(string=w435) -> (length=w442:i32)
                n161 = Greater?(x=w444, y=0) -> (0:w439:bool)
                n162 = Greater?(x=w442, y=0) -> (0:w440:bool)
                n163 = And(x=w440, y=w439) -> (x .and. y?=w438:bool)
                n164 = case shown="True" w438 {
                  tunnel: w437 -> [w445 w461]
                  tunnel: w436 -> [_ w448]
                  tunnel: w435 -> [_ w456]
                  tunnel: w434 -> [_ w457]
                  tunnel: [w445 w452] -> w433
                  tunnel: [_ w446] -> w432
                  frame False {
                  }
                  frame True {
                    w455 = T2."String" ("DataType")
                    w459 = "Config/Value/Value" ("MemberName")
                    # "Set SampleCount"
                    # "Set Freq 2"
                    # "Set Freq 1"
                    n165 = call "SetVariableConfig_Example.vi"("StringValue or Snippet 2"=w457, "Fehler (Eingang, kein Fehler)"=w461, "PropertyName"="General/Average/Frequency3dB1List", "DataType"=w455, "VariableID"=w448, "ConfigMemberName"=w459) -> ("Fehler (Ausgang)"=w458:errorcluster)  [unwired: 20 in, 1 out]
                    n166 = call "SetVariableConfig_Example.vi"("StringValue or Snippet 2"=w456, "Fehler (Eingang, kein Fehler)"=w458, "PropertyName"="General/Average/Frequency3dB2List", "DataType"=w455, "VariableID"=w448, "ConfigMemberName"=w459) -> ("Fehler (Ausgang)"=w453:errorcluster)  [unwired: 20 in, 1 out]
                    n167 = local read "SampleCount"() -> (w447:i64)
                    n168 = call "SetVariableConfig_Example.vi"("Int64Value"=w447, "Fehler (Eingang, kein Fehler)"=w453, "PropertyName"="General/Average/SampleCountRange", "DataType"=T2."Int64", "VariableID"=w448, "ConfigMemberName"="Config/Value" ("MemberName")) -> ("VariableInfo out"=w446:T3, "Fehler (Ausgang)"=w452:errorcluster)  [unwired: 20 in]
                  }
                }
              }
              frame "GrpHp" {
                # "High-Pass"
                n169 = String Length(string=w466) -> (length=w468:i32)
                n170 = Greater?(x=w468, y=0) -> (0:w465:bool)
                n171 = case shown="True" w465 {
                  tunnel: w471 -> [w476 w484]
                  tunnel: w469 -> [_ w479]
                  tunnel: w466 -> [_ w481]
                  tunnel: [w476 w478] -> w470
                  tunnel: [w472 w477] -> w464
                  tunnel: w463 -> [w475 _]
                  tunnel: w462 -> [w474 _]
                  frame False {
                    # "wirte old value"
                    n172 = Unbundle By Name(w474) -> ("Array"=w473:T3[])
                    n173 = Index Array(array=w473, index=w475) -> (element=w472:T3)
                  }
                  frame True {
                    # "Set Freq 1"
                    n174 = call "SetVariableConfig_Example.vi"("StringValue or Snippet 2"=w481, "Fehler (Eingang, kein Fehler)"=w484, "PropertyName"="General/Average/Frequency3dB1List", "DataType"=T2."String", "VariableID"=w479, "ConfigMemberName"="Config/Value/Value" ("MemberName")) -> ("VariableInfo out"=w477:T3, "Fehler (Ausgang)"=w478:errorcluster)  [unwired: 20 in]
                  }
                }
              }
              frame "GrpHpArMe" {
                # "High-Pass and Arithmetic mean"
                n175 = String Length(string=w489) -> (length=w491:i32)
                n176 = Greater?(x=w491, y=0) -> (0:w488:bool)
                n177 = case shown="True" w488 {
                  tunnel: w494 -> [w499 w512]
                  tunnel: w493 -> [_ w503]
                  tunnel: w489 -> [_ w509]
                  tunnel: [w499 w507] -> w492
                  tunnel: [w495 w500] -> w487
                  tunnel: w486 -> [w497 _]
                  tunnel: w485 -> [w496 _]
                  frame False {
                    # "wirte old value"
                    n178 = Unbundle By Name(w497) -> ("Array"=w498:T3[])
                    n179 = Index Array(array=w498, index=w496) -> (element=w495:T3)
                  }
                  frame True {
                    # "Set Freq 1"
                    n180 = call "SetVariableConfig_Example.vi"("StringValue or Snippet 2"=w509, "Fehler (Eingang, kein Fehler)"=w512, "PropertyName"="General/Average/Frequency3dB1List", "DataType"=T2."String", "VariableID"=w503, "ConfigMemberName"="Config/Value/Value" ("MemberName")) -> ("Fehler (Ausgang)"=w502:errorcluster)  [unwired: 20 in, 1 out]
                    n181 = local read "SampleCount"() -> (w501:i64)
                    n182 = call "SetVariableConfig_Example.vi"("Int64Value"=w501, "Fehler (Eingang, kein Fehler)"=w502, "PropertyName"="General/Average/SampleCountRange", "DataType"=T2."Int64", "VariableID"=w503, "ConfigMemberName"="Config/Value" ("MemberName")) -> ("VariableInfo out"=w500:T3, "Fehler (Ausgang)"=w507:errorcluster)  [unwired: 20 in]
                  }
                }
              }
              frame "GrpLp" {
                # "Low-Pass"
                n183 = String Length(string=w516) -> (length=w519:i32)
                n184 = Greater?(x=w519, y=0) -> (0:w517:bool)
                n185 = case shown="True" w517 {
                  tunnel: w522 -> [w527 w535]
                  tunnel: w521 -> [_ w530]
                  tunnel: w516 -> [_ w532]
                  tunnel: [w527 w529] -> w520
                  tunnel: [w523 w528] -> w515
                  tunnel: w514 -> [w525 _]
                  tunnel: w513 -> [w524 _]
                  frame False {
                    # "wirte old value"
                    n186 = Unbundle By Name(w525) -> ("Array"=w526:T3[])
                    n187 = Index Array(array=w526, index=w524) -> (element=w523:T3)
                  }
                  frame True {
                    # "Set Freq 1"
                    n188 = call "SetVariableConfig_Example.vi"("StringValue or Snippet 2"=w532, "Fehler (Eingang, kein Fehler)"=w535, "PropertyName"="General/Average/Frequency3dB1List", "DataType"=T2."String", "VariableID"=w530, "ConfigMemberName"="Config/Value/Value" ("MemberName")) -> ("VariableInfo out"=w528:T3, "Fehler (Ausgang)"=w529:errorcluster)  [unwired: 20 in]
                  }
                }
              }
              frame "GrpLpArMe" {
                # "Low-Pass and Arithmetic mean"
                n189 = String Length(string=w540) -> (length=w542:i32)
                n190 = Greater?(x=w542, y=0) -> (0:w539:bool)
                n191 = case shown="True" w539 {
                  tunnel: w545 -> [w550 w563]
                  tunnel: w544 -> [_ w554]
                  tunnel: w540 -> [_ w560]
                  tunnel: [w550 w558] -> w543
                  tunnel: [w546 w551] -> w538
                  tunnel: w537 -> [w548 _]
                  tunnel: w536 -> [w547 _]
                  frame False {
                    # "wirte old value"
                    n192 = Unbundle By Name(w548) -> ("Array"=w549:T3[])
                    n193 = Index Array(array=w549, index=w547) -> (element=w546:T3)
                  }
                  frame True {
                    # "Set Freq 1"
                    n194 = call "SetVariableConfig_Example.vi"("StringValue or Snippet 2"=w560, "Fehler (Eingang, kein Fehler)"=w563, "PropertyName"="General/Average/Frequency3dB1List", "DataType"=T2."String", "VariableID"=w554, "ConfigMemberName"="Config/Value/Value" ("MemberName")) -> ("Fehler (Ausgang)"=w553:errorcluster)  [unwired: 20 in, 1 out]
                    n195 = local read "SampleCount"() -> (w552:i64)
                    n196 = call "SetVariableConfig_Example.vi"("Int64Value"=w552, "Fehler (Eingang, kein Fehler)"=w553, "PropertyName"="General/Average/SampleCountRange", "DataType"=T2."Int64", "VariableID"=w554, "ConfigMemberName"="Config/Value" ("MemberName")) -> ("VariableInfo out"=w551:T3, "Fehler (Ausgang)"=w558:errorcluster)  [unwired: 20 in]
                  }
                }
              }
              frame "GrpBp" {
                # "Band-Pass"
                n197 = String Length(string=w567) -> (length=w575:i32)
                n198 = String Length(string=w568) -> (length=w573:i32)
                n199 = Greater?(x=w575, y=0) -> (0:w570:bool)
                n200 = Greater?(x=w573, y=0) -> (0:w571:bool)
                n201 = And(x=w571, y=w570) -> (x .and. y?=w569:bool)
                n202 = case shown="True" w569 {
                  tunnel: w578 -> [w583 w594]
                  tunnel: w577 -> [_ w586]
                  tunnel: w567 -> [_ w589]
                  tunnel: w568 -> [_ w590]
                  tunnel: [w583 w585] -> w576
                  tunnel: [w579 w584] -> w566
                  tunnel: w565 -> [w581 _]
                  tunnel: w564 -> [w580 _]
                  frame False {
                    # "wirte old value"
                    n203 = Unbundle By Name(w581) -> ("Array"=w582:T3[])
                    n204 = Index Array(array=w582, index=w580) -> (element=w579:T3)
                  }
                  frame True {
                    w588 = T2."String" ("DataType")
                    w592 = "Config/Value/Value" ("MemberName")
                    # "Set Freq 2"
                    # "Set Freq 1"
                    n205 = call "SetVariableConfig_Example.vi"("StringValue or Snippet 2"=w590, "Fehler (Eingang, kein Fehler)"=w594, "PropertyName"="General/Average/Frequency3dB1List", "DataType"=w588, "VariableID"=w586, "ConfigMemberName"=w592) -> ("Fehler (Ausgang)"=w591:errorcluster)  [unwired: 20 in, 1 out]
                    n206 = call "SetVariableConfig_Example.vi"("StringValue or Snippet 2"=w589, "Fehler (Eingang, kein Fehler)"=w591, "PropertyName"="General/Average/Frequency3dB2List", "DataType"=w588, "VariableID"=w586, "ConfigMemberName"=w592) -> ("VariableInfo out"=w584:T3, "Fehler (Ausgang)"=w585:errorcluster)  [unwired: 20 in]
                  }
                }
              }
            }
            n207 = Unbundle By Name(w399) -> ("Array"=w404:T3[])
            n208 = Replace Array Subset(array=w404, new element=w403, index=w400) -> (w402:T3[])
            n209 = Bundle By Name(cluster=w399, "Array"=w402) -> (w401:T4)
          }
        }
      }
    }
    n210 = Unbundle By Name(w28) -> ("status"=w17:bool)
    n211 = Wait Until Next ms Multiple(millisecond multiple=u32 100 ("Vielfache von ms")) -> ()  [unwired: 1 out]
    n212 = call <vilib>:"Simple Error Handler.vi"("error in (no error)"=w28) -> ()  [unwired: 1 in, 8 out]
  }
  n213 = property class="VI"(reference=w3, error in=w4, "Front Panel.Open"=FALSE ("Frontpanel-Fenster:Öffnen")) -> (error out=→"error out":errorcluster)  [unwired: 1 out]
